vi "Write Event Type.vi"(8 "error in (no error)":errorcluster, 10 "Event Type":T1, 11 "Dqmh Event in":refnum<class "Dqmh Event.lvclass">) -> (0 "error out":errorcluster, 3 "Dqmh Event out":refnum<class "Dqmh Event.lvclass">)   [LabVIEW 2021, in "TAF Proj Document Type.lvlib" / "Dqmh Event.lvclass"]
uses:
  <vilib>/Wovalab/AntiDoc/Document Type/Add-ons/LabVIEW TAF Project/Dqmh Event/Dqmh Event.lvclass
  <vilib>/Wovalab/AntiDoc/Document Type/Add-ons/LabVIEW TAF Project/Project Parser/Dqmh Event Type--enum.ctl
  <vilib>/Wovalab/AntiDoc/Document Type/Add-ons/LabVIEW TAF Project/Dqmh Event/Dqmh Event.lvclass/Dqmh Event.ctl
  <vilib>/Wovalab/AntiDoc/Document Type/Add-ons/LabVIEW TAF Project/Project Parser/Project Parser.lvlib
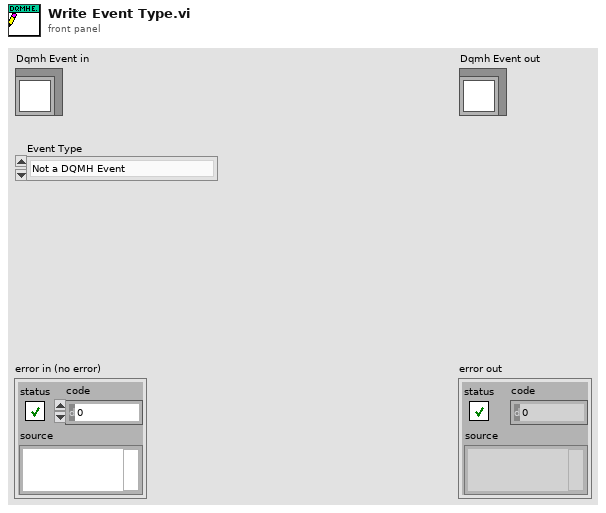
[diagram p1: front panel]
types:
  T1 = typedef "TAF Proj Document Type.lvlib/Project Parser.lvlib/Dqmh Event Type--enum.ctl" = enum16{"Not a DQMH Event", "Request", "Request And Wait For Reply", "Broadcast"}
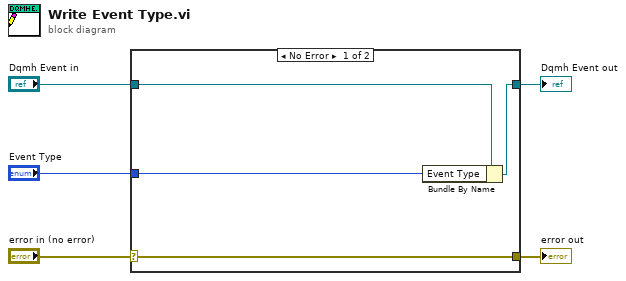
[diagram p0: block diagram]
diagram:
  n1 = case shown="No Error" "error in (no error)" {
    selector: "error in (no error)" -> [w9 w10]
    tunnel: [w9 w10] -> w4
    tunnel: [w7 w11] -> w2
    tunnel: "Dqmh Event in" -> [w8 w11]
    tunnel: "Event Type" -> [w6 _]
    frame No Error {
      n2 = Bundle By Name(cluster=w8, "Event Type"=w6) -> (w7:refnum<class "Dqmh Event.lvclass">)
    }
    frame Error {
    }
  }
  "error out" <- w4
  "Dqmh Event out" <- w2
